vi "AddNewBuv.vi"(0 "Num of Buvs in":u8, 2 "New BuV IP":string, 5 "Voltage":string, 7 "error in":errorcluster, 8 "Name Arr IN":string[](array[string]), 9 "New BuV name":string, 10 "Buv IP arr":string[](array[string]), 13 "BuvCtrlVI_VIRef":refnum<vi>[](array[refnum])) -> (12 "BuvCtrlVI_VIRefOut":refnum<vi>[](array[refnum]), 20 "Num of Buvs out":u8, 22 "Name Out":string[](array[string]), 24 "Buv Ip Out":string[](array[string]), 27 "error out":errorcluster)   [LabVIEW 2013]
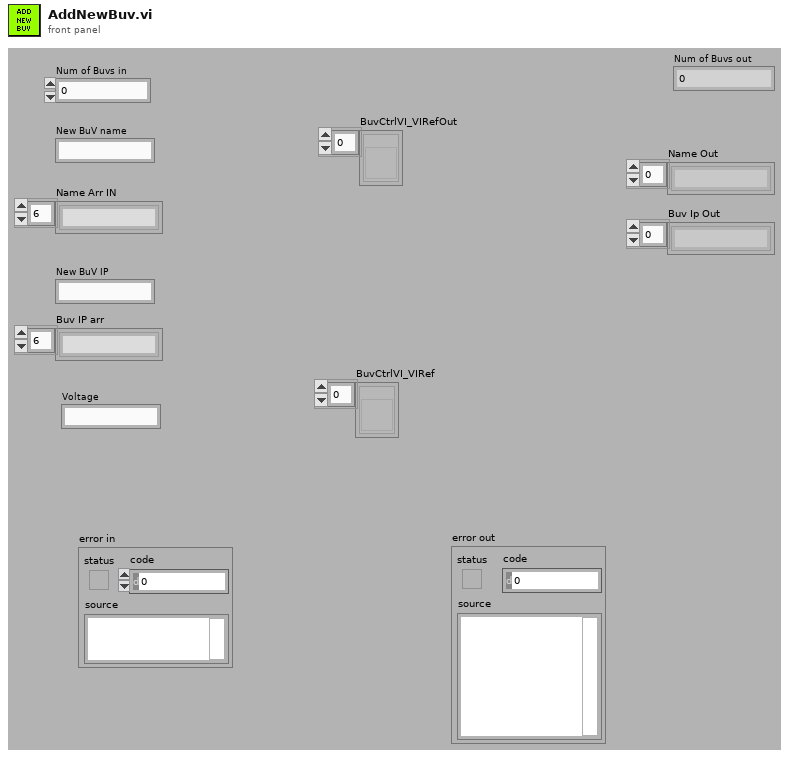
[diagram p1: front panel]
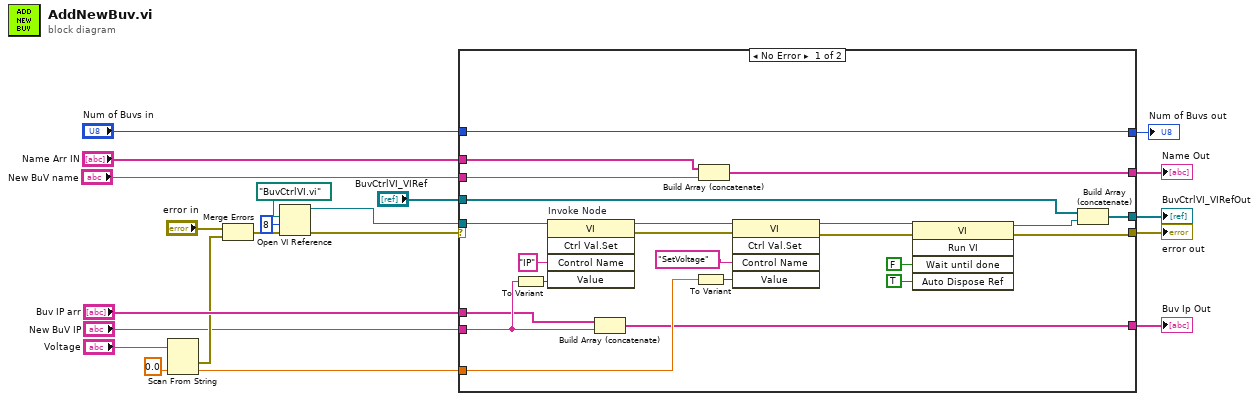
[diagram p0: block diagram]
diagram:
  n1 = Scan From String(input string="Voltage", default 1=0.0 ("default value 1")) -> (error out=w9:errorcluster, output 1=w15:dbl)  [unwired: 3 in, 2 out]
  n2 = Merge Errors("error in", w9) -> (w14:errorcluster)
  n3 = Open VI Reference(vi path=path "BuvCtrlVI.vi", options=8, error in (no error)=w14) -> (vi reference=w6:refnum<vi>, error out=w7:errorcluster)  [unwired: 1 in, 2 out]
  n4 = case shown="No Error" w7 {
    selector: w7 -> [_ w49]
    tunnel: w6 -> [w43 _]
    tunnel: [w23 w48] -> w19
    tunnel: [w28 w49] -> w18
    tunnel: "BuvCtrlVI_VIRef" -> [w24 w48]
    tunnel: "New BuV IP" -> [w37 _]
    tunnel: w15 -> [w36 _]
    tunnel: "Buv IP arr" -> [w35 w47]
    tunnel: [w34 w47] -> w12
    tunnel: "Name Arr IN" -> [w27 w46]
    tunnel: [w33 w46] -> w10
    tunnel: "New BuV name" -> [w26 _]
    tunnel: [w25 w45] -> w1
    tunnel: "Num of Buvs in" -> [w25 w45]
    frame No Error {
      n5 = To Variant(anything=w37) -> (Variant=w38:variant)
      n6 = invoke on="Invoke Node" class="VI" method="Ctrl Val.Set"(reference=w43, "Control Name"="IP", "Value"=w38) -> (reference out=w40:refnum<vi>, error out=w39:errorcluster)  [unwired: 2 in, 3 out]
      n7 = Build Array (concatenate)(w35, w37) -> (w34:string[])
      n8 = To Variant(anything=w36) -> (Variant=w41:variant)
      n9 = Build Array (concatenate)(w27, w26) -> (w33:string[])
      n10 = invoke class="VI" method="Ctrl Val.Set"(reference=w40, error in=w39, "Control Name"="SetVoltage", "Value"=w41) -> (reference out=w30:refnum<vi>, error out=w29:errorcluster)  [unwired: 1 in, 3 out]
      n11 = invoke class="VI" method="Run VI"(reference=w30, error in=w29, "Wait until done"=FALSE ("Wait Until Done"), "Auto Dispose Ref"=TRUE ("Auto Dispose Reference")) -> (reference out=w22:refnum<vi>, error out=w28:errorcluster)  [unwired: 1 in, 3 out]
      n12 = Build Array (concatenate)(w24, w22) -> (w23:refnum<vi>[])
    }
    frame Error {
    }
  }
  "error out" <- w18
  "BuvCtrlVI_VIRefOut" <- w19
  "Buv Ip Out" <- w12
  "Name Out" <- w10
  "Num of Buvs out" <- w1
